vi "分析光源均勻度.vi"(7 "ShowData":bool, 8 "error in (no error)":errorcluster, 10 "DieArea":i32 min=10, 11 "Image In":T1) -> (0 "error out":errorcluster, 3 "Image":T1(plugin-control))   [LabVIEW 2015]
uses:
  <vilib>/vision/Image Controls.llb/IMAQ Image.ctl
  <vilib>/vision/NI_Vision_Development_Module.lvlib
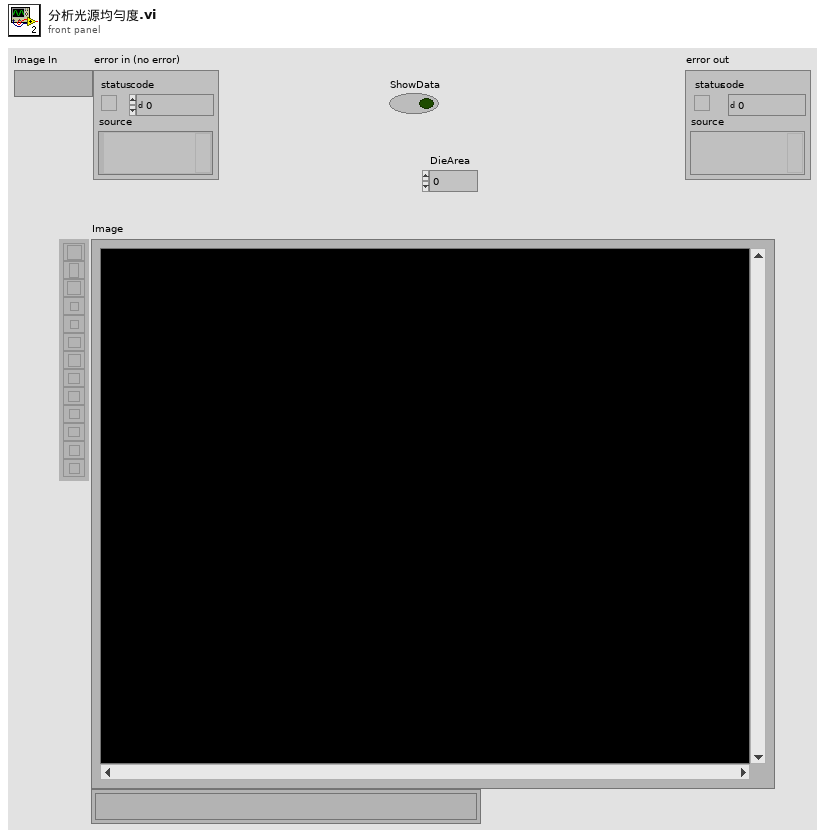
[diagram p1: front panel]
types:
  T1 = typedef "IMAQ Image.ctl" = refnum<image>
  T2 = cluster{"Left":i32, "Top":i32, "Right":i32, "Bottom":i32}
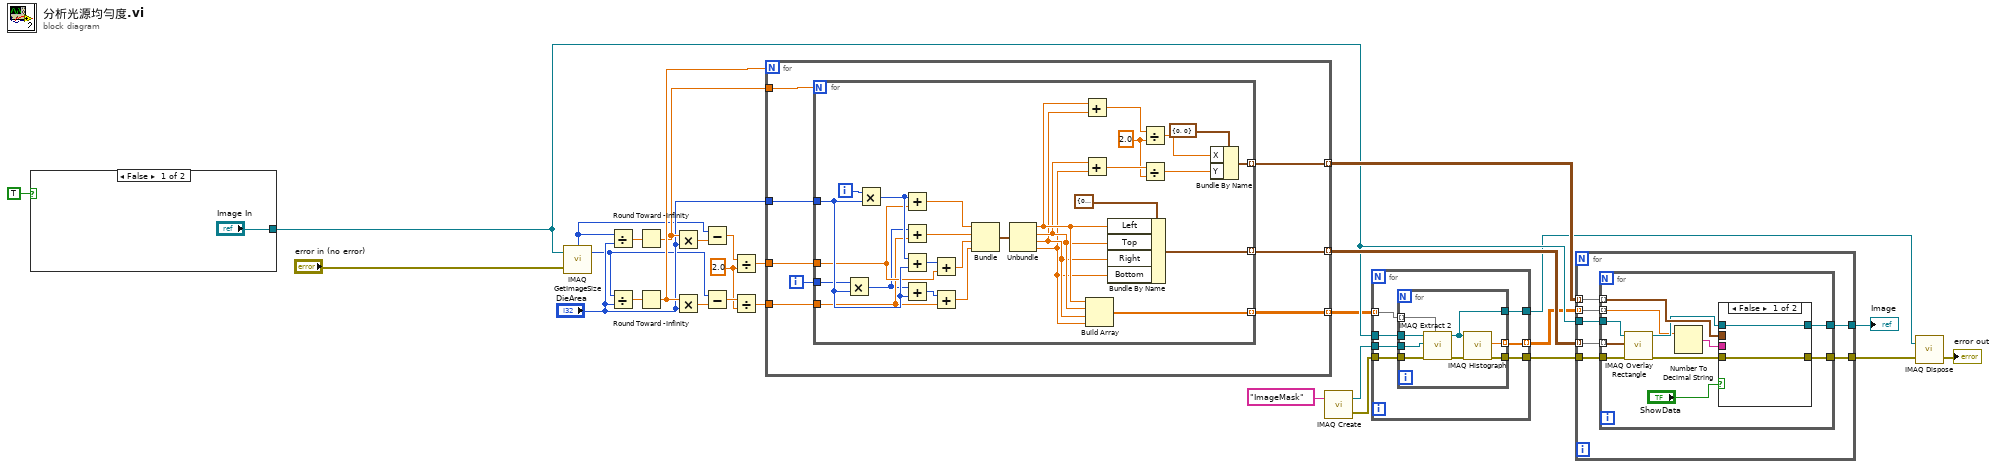
[diagram p0: block diagram]
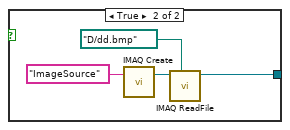
[diagram p2: hidden frame]
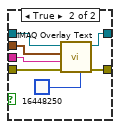
[diagram p3: hidden frame]
diagram:
  w5 = 2.0 ("y")
  n1 = case shown="False" TRUE {
    tunnel: ["Image In" w32] -> w24
    frame False {
    }
    frame True {
      n2 = call "IMAQ Create"("Image Name"="ImageSource") -> ("New Image"=w34:T1)  [unwired: 4 in, 1 out]
      n3 = call "IMAQ ReadFile"("File Path"=path "D:/dd.bmp", "Image"=w34) -> ("Image Out"=w32:T1)  [unwired: 5 in, 4 out]
    }
  }
  n4 = call "IMAQ GetImageSize"("Image"=w24, "error in (no error)"="error in (no error)") -> ("Y Resolution"=w10:i32, "X Resolution"=w4:i32)  [unwired: 2 in, 1 out]
  n5 = Divide(x=w4, y="DieArea") -> (x/y=w29:dbl)
  n6 = Divide(x=w10, y="DieArea") -> (x/y=w28:dbl)
  n7 = Round Toward -Infinity(1:w29) -> (0:w12:dbl)
  n8 = Round Toward -Infinity(1:w28) -> (0:w13:dbl)
  n9 = Multiply(x=w12, y="DieArea") -> (x*y=w8:dbl)
  n10 = Multiply(x=w13, y="DieArea") -> (x*y=w9:dbl)
  n11 = Subtract(x=w4, y=w8) -> (x-y=w6:dbl)
  n12 = Subtract(x=w10, y=w9) -> (x-y=w7:dbl)
  n13 = Divide(x=w6, y=w5) -> (x/y=w3:dbl)
  n14 = Divide(x=w7, y=w5) -> (x/y=w2:dbl)
  n15 = for {
    N: w13 -> [_]
    tunnel: w12 -> [w42]
    tunnel: "DieArea" -> [w41]
    tunnel: [w40] -> w26 mode=indexing
    tunnel: [w39] -> w27 mode=indexing
    tunnel: [w38] -> w21 mode=indexing
    tunnel: w3 -> [w37]
    tunnel: w2 -> [w35]
    i -> [w36]
    n16 = for {
      N: w42 -> [_]
      tunnel: w36 -> [w68]
      tunnel: w41 -> [w70]
      tunnel: [w66] -> w40 mode=indexing
      tunnel: [w65] -> w39 mode=indexing
      tunnel: [w64] -> w38 mode=indexing
      tunnel: w37 -> [w50]
      tunnel: w35 -> [w47]
      i -> [w58]
      w61 = 2.0 ("y")
      n17 = Multiply(x=w68, y=w70) -> (x*y=w46:i32)
      n18 = Multiply(x=w58, y=w70) -> (x*y=w52:i32)
      n19 = Add(x=w52, y=w50) -> (x+y=w51:dbl)
      n20 = Add(x=w46, y=w47) -> (x+y=w45:dbl)
      n21 = Add(x=w52, y=w70) -> (x+y=w49:i32)
      n22 = Add(x=w46, y=w70) -> (x+y=w44:i32)
      n23 = Add(x=w49, y=w50) -> (x+y=w48:dbl)
      n24 = Add(x=w44, y=w47) -> (x+y=w43:dbl)
      n25 = Bundle(w51, w45, w48, w43) -> (w57:cluster{dbl, dbl, dbl, dbl})  [unwired: 1 in]
      n26 = Unbundle(w57) -> (w56:dbl, w55:dbl, w54:dbl, w53:dbl)
      n27 = Add(x=w56, y=w54) -> (x+y=w62:dbl)
      n28 = Add(x=w55, y=w53) -> (x+y=w63:dbl)
      n29 = Build Array(w56, w55, w54, w53) -> (w64:dbl[])
      n30 = Bundle By Name(cluster=T2 {"Left"=0, "Top"=0, "Right"=0, "Bottom"=0} ("Rectangle"), "Left"=w56, "Top"=w55, "Right"=w54, "Bottom"=w53) -> (w66:T2)
      n31 = Divide(x=w62, y=w61) -> (x/y=w59:dbl)
      n32 = Divide(x=w63, y=w61) -> (x/y=w60:dbl)
      n33 = Bundle By Name(cluster=cluster{"X":i32, "Y":i32} {"X"=0, "Y"=0} ("Origin"), "X"=w59, "Y"=w60) -> (w65:cluster{"X":i32, "Y":i32})
    }
  }
  n34 = call "IMAQ Create"("Image Name"="ImageMask") -> ("New Image"=w22:T1, "error out"=w18:errorcluster)  [unwired: 4 in]
  n35 = for {
    tunnel: w24 -> [w77]
    tunnel: w22 -> [w76]
    tunnel: w21 -> [w75] mode=indexing
    tunnel: [w74] -> w20 mode=indexing
    tunnel: w18 -> [w73]
    tunnel: [w72] -> w17
    tunnel: [w71] -> w1
    n36 = for {
      tunnel: w77 -> [w83]
      tunnel: w76 -> [w84]
      tunnel: w75 -> [w85] mode=indexing
      tunnel: [w82] -> w74 mode=indexing
      tunnel: w73 -> [w81]
      tunnel: [w79] -> w72
      tunnel: [w78] -> w71
      n37 = call "IMAQ Extract 2"("Optional Rectangle"=w85, "error in (no error)"=w81, "Image Dst"=w84, "Image Src"=w83) -> ("error out"=w80:errorcluster, "Image Dst Out"=w78:T1)  [unwired: 6 in]
      n38 = call "IMAQ Histograph"("error in (no error)"=w80, "Image"=w78) -> ("error out"=w79:errorcluster, "Mean Value"=w82:sgl)  [unwired: 6 in, 2 out]
    }
  }
  n39 = for {
    tunnel: w27 -> [w92] mode=indexing
    tunnel: w26 -> [w91] mode=indexing
    tunnel: w24 -> [w90]
    tunnel: [w89] -> w25
    tunnel: w20 -> [w88] mode=indexing
    tunnel: w17 -> [w87]
    tunnel: [w86] -> w16
    n40 = for {
      tunnel: w92 -> [w103] mode=indexing
      tunnel: w91 -> [w102] mode=indexing
      tunnel: w90 -> [w101]
      tunnel: [w99] -> w89
      tunnel: w88 -> [w98] mode=indexing
      tunnel: w87 -> [w96]
      tunnel: [w94] -> w86
      n41 = call "IMAQ Overlay Rectangle"("error in (no error)"=w96, "Rectangle"=w102, "Image"=w101) -> ("error out"=w95:errorcluster, "Image Out"=w100:T1)  [unwired: 7 in]
      n42 = Number To Decimal String(number=w98) -> (decimal integer string=w97:string)  [unwired: 1 in]
      n43 = case shown="False" "ShowData" {
        tunnel: w103 -> [_ w112]
        tunnel: w100 -> [w104 w111]
        tunnel: [w104 w110] -> w99
        tunnel: w97 -> [_ w109]
        tunnel: w95 -> [w105 w108]
        tunnel: [w105 w107] -> w94
        frame False {
        }
        frame True {
          n44 = call "IMAQ Overlay Text"("BG Color (Transparent)"=u32 16448250, "error in (no error)"=w108, "String"=w109, "Origin"=w112, "Image"=w111) -> ("error out"=w107:errorcluster, "Image Out"=w110:T1)  [unwired: 5 in]
        }
      }
    }
  }
  "Image" <- w25
  n45 = call "IMAQ Dispose"("Image"=w1, "error in (no error)"=w16) -> ("error out"=→"error out":errorcluster)  [unwired: 4 in]
